vi "Example.vi"() -> ()   [LabVIEW 2014, in "Stanford Research DG645 - Driver.lvlib"]
uses:
  Stanford Research DG645 - Driver.lvlib
  Driver/Output BNC.ctl
  Driver/Channel.ctl
  Driver/Polarity.ctl
panel:
  in  "Main Tab Control":T1(tab)
  in  "Common IEEE-488.2 Tab Control":T2(tab)
  in  "Calibrate":bool
  out "Calibration Result Code":i32
  out "Auto Calibration passed succesfully":bool
  in  "Clear Status":bool
  out "Current ESE Register":i32
  in  "get ESE":bool
  in  "Set ESE Register":i32
  in  "get Event Status Register":bool
  out "Current Event Status Register Values":T3
  out "Current ESR Register":i32
  in  "Identify Device":bool
  out "Model":string
  out "Instrument Firmware Revision":string
  out "Complete Answer String":string
  out "Manufacturer":string
  out "Serial Number":string
  out "Operation complete?":bool
  out "Current Operation Comlete":i32
  in  "get Operation Complete":bool
  in  "set Operation Complete":bool
  out "Current PSC flag":bool
  in  "get PSC flag":bool
  in  "Set PSC flag":bool
  in  "Recall Settings":i32
  in  "Reset":bool
  in  "Save Settings":i32
  out "Current SRE":i32
  in  "get SRE":bool
  in  "Set SRE":i32
  in  "get Status Byte":bool
  out "Current Status Byte":i32
  out "Current Status Byte Register":T4
  in  "Trigger":bool
  in  "Self Test":bool
  out "Self-Test Result Code":i32
  out "Self Test passed succesfully":bool
  in  "Wait for Command Execution":bool
  in  "Status and Display":T5(tab)
  in  "Set Display Value":i32(ring) items=["Trigger rate", "Trigger threshold", "Trigger single shot", "Trigger line", "Advanced triggering enable", "Trigger holdoff", "Prescale configuration", "Burst mode", "Burst delay", "Burst count", "Burst period", "Channel delay", "Channel output levels", "Channel output polarity", "Burst T0 configuration"]
  in  "Set Channel":T6 items=["T0", "T1", "A", "B", "C", "D", "E", "F", "G", "H"]
  in  "Get Display":bool
  out "Current Display Value":i32(ring) items=["Trigger rate", "Trigger threshold", "Trigger single shot", "Trigger line", "Advanced triggering enable", "Trigger holdoff", "Prescale configuration", "Burst mode", "Burst delay", "Burst count", "Burst period", "Channel delay", "Channel output levels", "Channel output polarity", "Burst T0 configuration"]
  out "Current Channel":T6 items=["T0", "T1", "A", "B", "C", "D", "E", "F", "G", "H"]
  in  "Set INSE register":i32
  out "Current INSE register":i32
  in  "Get INSE register":bool
  in  "Get Instrument Status":bool
  out "Current Instrument Status Register Values":T7
  out "Current Instrument Status Register":i32
  in  "Get Error":bool
  in  "Set Show Display":bool
  out "Display shown?":bool
  in  "Get Show Display":bool
  in  "Get Timebase":bool
  out "Current Timebase":i32(ring) items=["Internal", "OCXO", "Rubidium", "External"]
  in  "Trigger":T8(tab)=enum."Step Holdoff"
  out "Adv. Trig. set?":bool
  in  "Set Adv. Triggering":bool
  in  "Get Adv. Triggering":bool
  out "Current Holdoff":dbl
  in  "Set Holdoff":dbl
  in  "Get Holdoff":bool
  in  "Set Inhibit":i32(ring) items=["Off", "Triggers", "AB", "AB and CD", "AB, CD and EF", "AB, CD, EF and GH"]
  in  "Get Inhibit":bool
  out "Current Trigger Inhibit State":i32(ring) items=["Off", "Triggers", "AB", "AB and CD", "AB, CD and EF", "AB, CD, EF and GH"]
  in  "Set Prescale Phase Factor":i32
  out "Current Prescale Phase Factor":i32
  in  "Prescaler to be set (PSPF)":i32(ring)=1 items=["Output AB"=1, "Output CD"=2, "Output EF"=3, "Output GH"=4]
  in  "Get Prescale Phase Factor":i32(ring)=1 items=["Output AB"=1, "Output CD"=2, "Output EF"=3, "Output GH"=4]
  in  "Set Prescale Factor":i32
  out "Current Prescale Factor":i32
  in  "Prescaler to be set (PSF)":i32(ring)=1 items=["Output AB"=1, "Output CD"=2, "Output EF"=3, "Output GH"=4]
  in  "Get Prescale Factor":i32(ring)=1 items=["Output AB"=1, "Output CD"=2, "Output EF"=3, "Output GH"=4]
  out "Step Size Holdoff [s]":dbl
  in  "Set Step Size Holdoff [s]":dbl
  in  "Holdoff Step Direction":bool
  in  "Step Holdoff":bool
  in  "Get Step Size Holdoff":bool
  out "Step Size Prescale Phase":i32
  in  "Set Step Size Prescale Phase":i32
  in  "Prescale Phase Step Direction":bool
  in  "Step Prescale Phase":bool
  in  "Get Step Size Prescale Phase":bool
  in  "Prescaler PPF":i32(ring)=1 items=["Output AB"=1, "Output CD"=2, "Output EF"=3, "Output GH"=4]
  out "Step Size  Phase Factor":i32
  in  "Set Step Size  Phase Factor":i32
  in  "Phase Factor Step Direction":bool
  in  "Step Phase Factor":bool
  in  "Get Step Size  Phase Factor":bool
  in  "Prescaler PF":i32(ring)=1 items=["Output AB"=1, "Output CD"=2, "Output EF"=3, "Output GH"=4]
  out "Step Size Trig Level [V]":dbl
  in  "Set Step Size Trig Level [V]":dbl
  in  "Trig Level Step Direction":bool
  in  "Step Trig Level":bool
  in  "Get Step Size Trig Level":bool
  out "Step Size Trig Rate [Hz]":dbl
  in  "Set Step Size Trig Rate [Hz]":dbl
  in  "Trig Rate Step Direction":bool
  in  "Step Trig Rate":bool
  in  "Get Step Size Trig Rate":bool
  in  "Get Trigger Level":bool
  in  "Set Trigger Level [V]":dbl=1.0
  out "Current Trigger Level [V]":dbl
  in  "Get Trigger Rate":bool
  in  "Set Trigger Rate [Hz]":dbl=1000.0
  out "Current Trigger Rate [Hz]":dbl
  in  "Set Trigger Source":i32(ring) items=["Internal", "External rising edge", "External falling edge", "Single shot external rising edges", "Single shot external falling edges", "Single shot", "Line"]
  in  "Get Trigger Source":bool
  out "Current Trigger Source":i32(ring) items=["Internal", "External rising edge", "External falling edge", "Single shot external rising edges", "Single shot external falling edges", "Single shot", "Line"]
  in  "Burst":T9(tab)
  out "Current Burst Count":i32
  in  "Set Burst Count":i32
  in  "Get Burst Count":bool
  out "Current Burst Delay [s]":dbl
  in  "Set Burst Delay [s]":dbl
  in  "Get Burst Delay":bool
  in  "Set Burst Mode":bool
  in  "Get Burst Mode":bool
  out "Burst Mode enabled?":bool
  in  "Set Burst Period [s]":dbl
  in  "Get Burst Period":bool
  out "Current Burst Period [s]":dbl
  in  "Set Burst T0 Config":bool
  in  "Get Burst T0 Config":bool
  out "Burst T0 Config enabled?":bool
  in  "Burst Count Step Direction":bool
  in  "Set Burst Count Step Size":i32
  in  "Step Burst Count":bool
  in  "Get Burst Count Step Size":bool
  out "Burst Count Step Size":i32
  in  "Burst Delay Step Direction":bool
  in  "Set Burst Delay Step Size [s]":dbl
  in  "Step Burst Delay":bool
  in  "Get Burst Delay Step Size":bool
  out "Burst Delay Step Size [s]":dbl
  in  "Burst Period Step Direction":bool
  in  "Set Burst Period Step Size [Hz]":dbl
  in  "Step Burst Period":bool
  in  "Get Burst Period Step Size":bool
  out "Burst Period Step Size [Hz]":dbl
  in  "Delay and Output":T10(tab)=enum."Offset"
  in  "Set: relative to":T6 items=["T0", "T1", "A", "B", "C", "D", "E", "F", "G", "H"]
  in  "Set: Delay [s]":dbl
  in  "Set Delay Channel":T6 items=["T0", "T1", "A", "B", "C", "D", "E", "F", "G", "H"]
  in  "Get Delay Channel":T6 items=["T0", "T1", "A", "B", "C", "D", "E", "F", "G", "H"]
  out "currently relative to":T6 items=["T0", "T1", "A", "B", "C", "D", "E", "F", "G", "H"]
  out "Current Delay [s]":dbl
  in  "Set: Level Amplitude [V]":dbl
  in  "Set Level Amplitude Output BNC":T11 items=["T0", "AB", "CD", "EF", "GH"]
  in  "Get Level Amplitude Output BNC":T11 items=["T0", "AB", "CD", "EF", "GH"]
  out "Current Level Amplitude Output BNC [V]":dbl
  in  "Set: Link to":T6=3 items=["T0", "T1", "A", "B", "C", "D", "E", "F", "G", "H"]
  in  "Set Link of Channel":T6=2 items=["T0", "T1", "A", "B", "C", "D", "E", "F", "G", "H"]
  in  "Get Link of Channel":T6=2 items=["T0", "T1", "A", "B", "C", "D", "E", "F", "G", "H"]
  out "currently linked to":T6 items=["T0", "T1", "A", "B", "C", "D", "E", "F", "G", "H"]
  in  "Set Level Offset [V]":dbl=1.0
  in  "Set Level Offset of Output":T11 items=["T0", "AB", "CD", "EF", "GH"]
  in  "Get Level Offset of Output":T11 items=["T0", "AB", "CD", "EF", "GH"]
  out "Current Level Offset [V]":dbl
  in  "Set Level Polarity of Output":T11 items=["T0", "AB", "CD", "EF", "GH"]
  in  "Get Level Polarity of Output":T11 items=["T0", "AB", "CD", "EF", "GH"]
  out "Current Polarity":T12 items=["negative", "positive"]
  in  "Polarity to be set":T12=1 items=["negative", "positive"]
  in  "Set Step Size Delay [s]":dbl
  in  "Delay Step Direction":bool
  in  "Step Delay":bool
  out "Step Size Delay [s]":dbl
  in  "Get Step Size Delay":bool
  in  "Channel Step Delay":T6 items=["T0", "T1", "A", "B", "C", "D", "E", "F", "G", "H"]
  in  "Set Step Size L-Amplitude [V]":dbl
  in  "Level Amplitude Step Direction":bool
  in  "Step Level Amplitude":bool
  out "Step Size  Level Amplitude [V]":dbl
  in  "Get Step Size Level Amplitude":bool
  in  "Output BNC Step Level Ampitude":T11 items=["T0", "AB", "CD", "EF", "GH"]
  in  "Set Step Size L-Offset [V]":dbl
  in  "Level Offset Step Direction":bool
  in  "Step Level Offset":bool
  out "Step Size  Level Offset [V]":dbl
  in  "Get Step Size Level Offset":bool
  in  "Output BNC Level Offset":T11 items=["T0", "AB", "CD", "EF", "GH"]
  in  "Interface":T13(tab)=enum."Interface Config"
  in  "Get Ethernet MAC Address":bool
  out "Ethernet MAC address":string="\r\n"
  out "Ethernet Physical Layer Config":bool
  in  "Get Ethernet Physical Layer Config":i32(ring) items=["Enable/disable Auto-negotiation of link speed", "Set link speed to 10 Base-T or 100 Base T"]
  in  "Set Ethernet Physical Layer Config":i32(ring) items=["Enable/disable Auto-negotiation of link speed", "Set link speed to 10 Base-T or 100 Base T"]
  in  "Ethernet Physical Layer Config to set":bool
  in  "Get Interface Config":i32(ring) items=["RS-232 Enable/Disable", "RS-232 Baud Rate", "GPIB Enable/Disable", "GPIB Address", "LAN TCP/IP Enable/Disable", "DHCP Enable/Disable", "Auto-Ip Enable/Disable", "Static Ip Enable/Disable", "Bare Socket Enable/Disable", "Telnet Enable/Disable", "VXI-11 Net Instrument Enable/Disable", "Static IP Address", "Subnet Address/Network Mask", "Default Gateway"]
  out "Current Interface Config Value":string
  in  "Set Interface Config":i32(ring) items=["RS-232 Enable/Disable", "RS-232 Baud Rate", "GPIB Enable/Disable", "GPIB Address", "LAN TCP/IP Enable/Disable", "DHCP Enable/Disable", "Auto-Ip Enable/Disable", "Static Ip Enable/Disable", "Bare Socket Enable/Disable", "Telnet Enable/Disable", "VXI-11 Net Instrument Enable/Disable", "Static IP Address", "Subnet Address/Network Mask", "Default Gateway"]
  in  "Interface Config Value to set":string
  in  "Interface to reset":i32(ring) items=["RS-232", "GPIB", "LAN TCP/IP"]
  in  "Set Local":bool
  in  "Set Remote":bool
  in  "Lock":bool
  out "locked?":bool
  out "unlocked?":bool
  in  "Unlock":bool
  in  "i":i32
  in  "j":i32
  in  "k":i32
  in  "Utility":enum32{"Revision"}(tab)
  in  "Get Revision":bool
  out "Instrument Driver Revision":string
  out "Instrument Firmware Rev":string
  out "Device Errors":cluster{"code":i32, "Text":string}[](array[cluster])
  in  "stop":bool
  out "error out":errorcluster
  in  "VISA resource name":refnum<visa-resource-name>
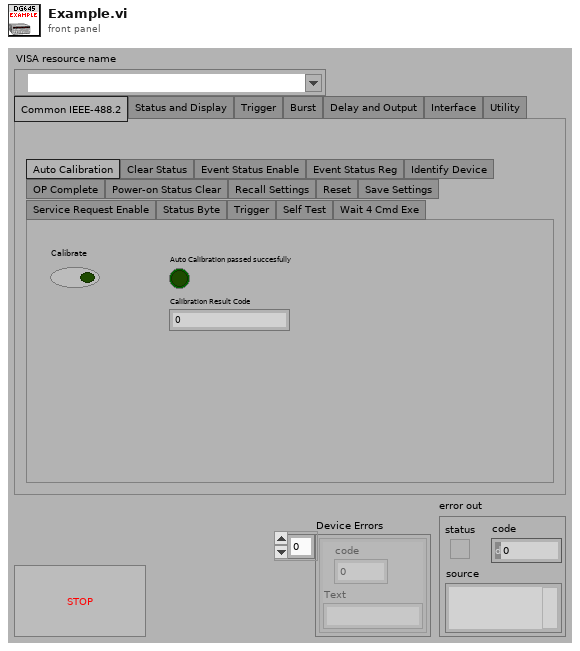
[diagram p1: front panel]
types:
  T1 = enum32{"Common IEEE-488.2", "Status and Display", "Trigger", "Burst", "Delay and Output", "Interface", "Utility"}
  T2 = enum32{"Auto Calibration", "Clear Status", "Event Status Enable", "Event Status Reg", "Identify Device", "OP Complete", "Power-on Status Clear", "Recall Settings", "Reset", "Save Settings", "Service Request Enable", "Status Byte", "Trigger", "Self Test", "Wait 4 Cmd Exe"}
  T3 = cluster{"Operation complete":bool, "reserved":bool, "Query Error":bool, "Device dependent Error":bool, "Execution Error":bool, "Command Error":bool, "reserved 2":bool, "Power-On":bool}
  T4 = cluster{"INSR Summary Bit":bool, "BUSY":bool, "reserved":bool, "reserved 2":bool, "message available":bool, "ESR Summary Bit":bool, "Master Summary Bit":bool, "reserved 3":bool}
  T5 = enum32{"Display", "Instrument Status Enable", "Instrument Status", "Error", "Show Display", "Timebase"}
  T6 = typedef "Stanford Research DG645 - Driver.lvlib/Channel.ctl" = i32
  T7 = cluster{"Got a trigger":bool, "Got a trigger while a delay or burst was in progress":bool, "a delay cycle has completed":bool, "a burst cycle has completed":bool, "a trigger or output delay cycle was inhibited":bool, "a delay cycle was aborted early":bool, "the 100MHz PLL came unlocked":bool, "the installed Rb oscillator is unlocked":bool}
  T8 = enum32{"Adv. Trig.", "Holdoff", "Inhibit", "Prescale Phase", "Prescale", "Step Holdoff", "Step PPF", "Step PF", "Step Trig Level", "Step Trig Rate", "Trig Level", "Trig Rate", "Trig Source"}
  T9 = enum32{"Count", "Delay", "Mode", "Period", "T0 Config", "Step Burst Count", "Step Burst Delay", "Step Bur Per"}
  T10 = enum32{"Delay", "Amplitude", "Link Channel", "Offset", "Polarity", "Step Delay", "Step Amplitude", "Step Offset"}
  T11 = typedef "Stanford Research DG645 - Driver.lvlib/Output BNC.ctl" = i32
  T12 = typedef "Stanford Research DG645 - Driver.lvlib/Polarity.ctl" = i32
  T13 = enum32{"MAC", "Ethernet Config", "Interface Config", "Interface Reset", "Local/Remote", "Lock/Unlock", "Term"}
  T14 = typedef "Stanford Research DG645.lvlib/Channel.ctl" = i32
  T15 = typedef "Stanford Research DG645.lvlib/Output BNC.ctl" = i32
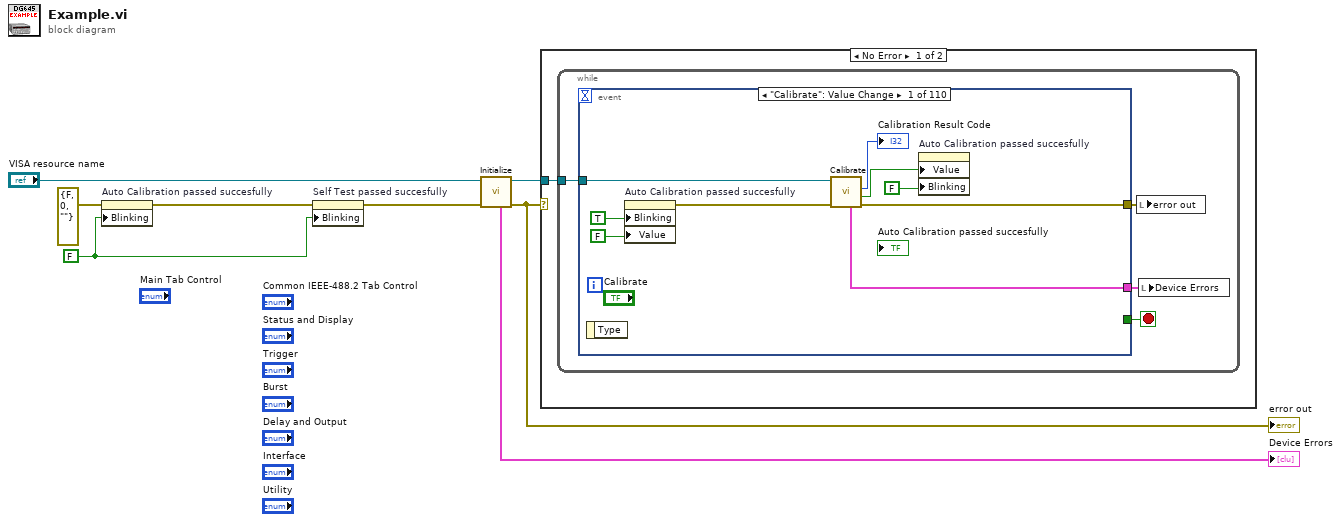
[diagram p0: block diagram]
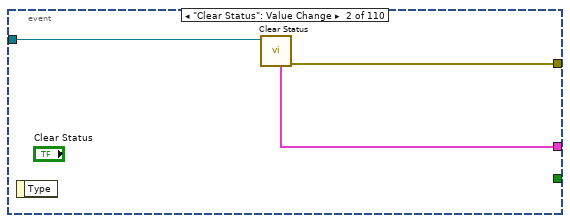
[diagram p2: hidden frame]
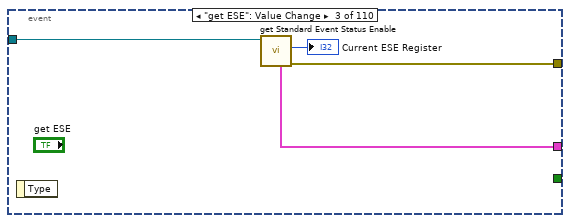
[diagram p3: hidden frame]
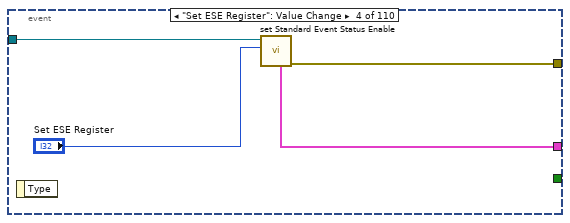
[diagram p4: hidden frame]
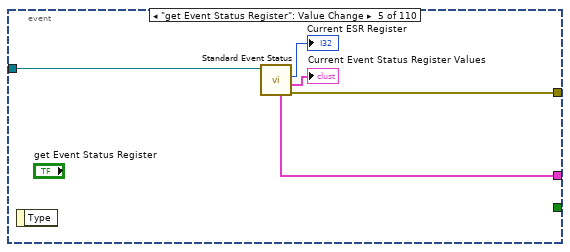
[diagram p5: hidden frame]
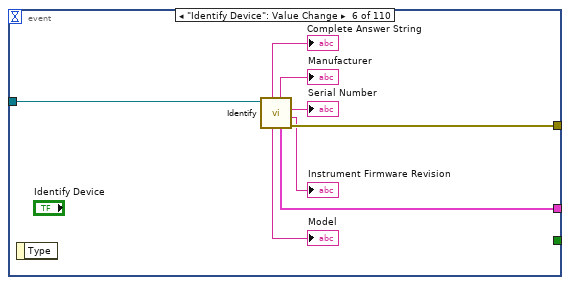
[diagram p6: hidden frame]
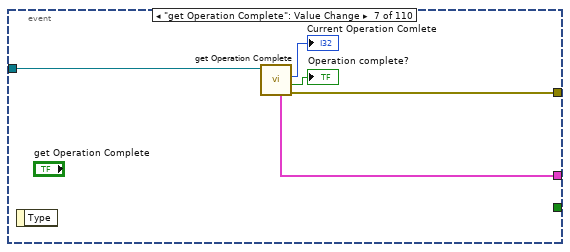
[diagram p7: hidden frame]
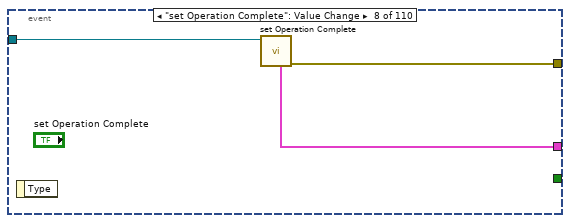
[diagram p8: hidden frame]
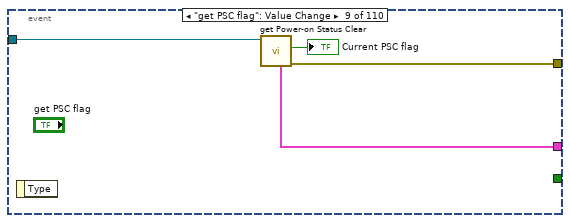
[diagram p9: hidden frame]
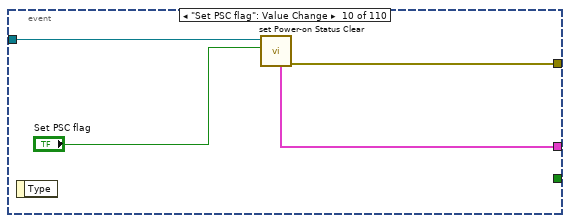
[diagram p10: hidden frame]
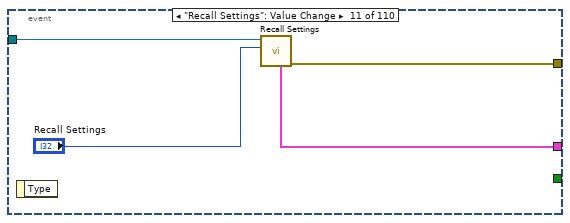
[diagram p11: hidden frame]
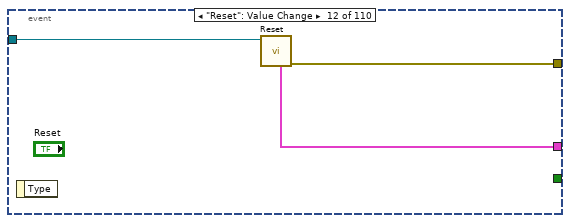
[diagram p12: hidden frame]
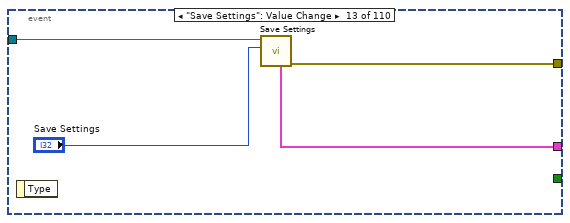
[diagram p13: hidden frame]
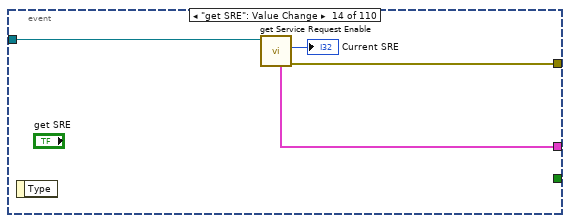
[diagram p14: hidden frame]
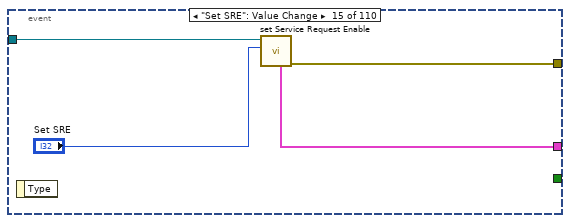
[diagram p15: hidden frame]
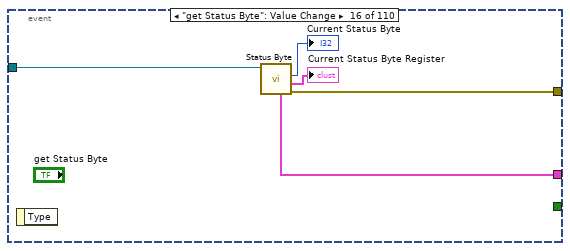
[diagram p16: hidden frame]
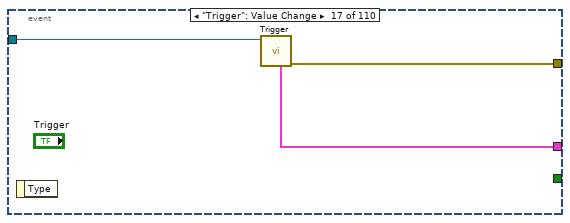
[diagram p17: hidden frame]
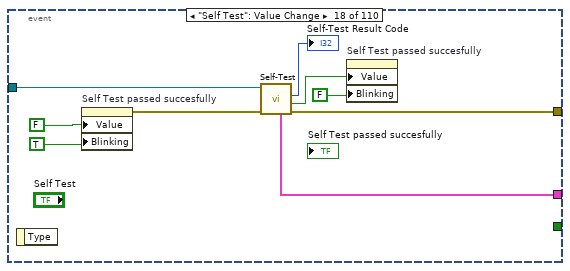
[diagram p18: hidden frame]
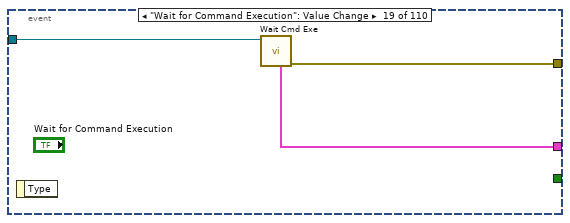
[diagram p19: hidden frame]
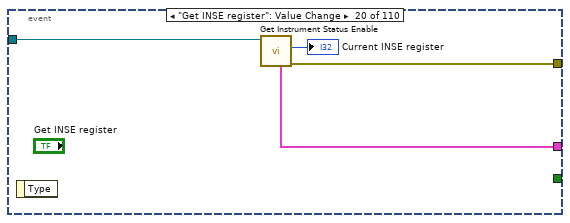
[diagram p20: hidden frame]
diagram:
  w1 = FALSE
  n1 = property on="Auto Calibration passed succesfully" class="Bool (strict)"(error in=errorcluster {"status"=FALSE, "code"=0, "source"=""} ("error out"), "Blinking"=w1) -> (error out=w4:errorcluster)  [unwired: 1 in, 1 out]
  n2 = property on="Self Test passed succesfully" class="Bool (strict)"(error in=w4, "Blinking"=w1) -> (error out=w2:errorcluster)  [unwired: 1 in, 1 out]
  n3 = call "Initialize.vi"("error in (no error)"=w2, "VISA resource name"="VISA resource name") -> ("error out"=w6:errorcluster, "VISA resource name out"=w7:refnum<visa-resource-name>, "Device Errors"=→"Device Errors":cluster{"code":i32, "Text":string}[])  [unwired: 7 in]
  "error out" <- w6
  n4 = case shown="No Error" w6 {
    tunnel: w7 -> [w9 _]
    frame No Error {
      n5 = while {
        tunnel: w9 -> [w13]
        stop <- w12 stop-if-true
        n6 = event shown="[0] \"Calibrate\": Value Change" {
          selector: _ -> [_ _ _ _ _ _ _ _ _ _ _ _ _ _ _ _ _ _ _ _ _ _ _ _ _ _ _ _ _ _ _ _ _ _ _ _ _ _ _ _ _ _ _ _ _ _ _ _ _ _ _ _ _ _ _ _ _ _ _ _ _ _ _ _ _ _ _ _ _ _ _ _ _ _ _ _ _ _ _ _ _ _ _ _ _ _ _ _ _ _ _ _ _ _ _ _ _ _ _ _ _ _ _ _ _ _ _ _ _ _]
          dyn-events: _ -> [_ _ _ _ _ _ _ _ _ _ _ _ _ _ _ _ _ _ _ _ _ _ _ _ _ _ _ _ _ _ _ _ _ _ _ _ _ _ _ _ _ _ _ _ _ _ _ _ _ _ _ _ _ _ _ _ _ _ _ _ _ _ _ _ _ _ _ _ _ _ _ _ _ _ _ _ _ _ _ _ _ _ _ _ _ _ _ _ _ _ _ _ _ _ _ _ _ _ _ _ _ _ _ _ _ _ _ _ _ _]
          timeout: _ -> [_ _ _ _ _ _ _ _ _ _ _ _ _ _ _ _ _ _ _ _ _ _ _ _ _ _ _ _ _ _ _ _ _ _ _ _ _ _ _ _ _ _ _ _ _ _ _ _ _ _ _ _ _ _ _ _ _ _ _ _ _ _ _ _ _ _ _ _ _ _ _ _ _ _ _ _ _ _ _ _ _ _ _ _ _ _ _ _ _ _ _ _ _ _ _ _ _ _ _ _ _ _ _ _ _ _ _ _ _ _]
          tunnel: [w14 w25 w29 w33 w38 w46 w51 w54 w58 w62 w66 w69 w73 w77 w81 w86 w87 w90 w99 w103 w108 w113 w117 w122 w127 w131 w135 w139 w143 w147 w151 w155 w159 w163 w168 w173 w177 w182 w186 w190 w194 w199 w205 w211 w216 w222 w228 w232 w236 w240 w244 w248 w252 w256 w260 w264 w268 w272 w276 w280 w284 w288 w292 w296 w300 w304 w308 w312 w316 w320 w324 w328 w332 w336 w340 w344 w348 w352 w358 w364 w369 w374 w379 w384 w389 w394 w399 w404 w409 w415 w421 w426 w432 w438 w443 w449 w455 w459 w464 w469 w474 w479 w483 w486 w490 w493 w497 w503 w508 w512] -> w11
          tunnel: w13 -> [w22 w24 w28 w32 w37 w45 w50 w53 w57 w61 w65 w68 w72 w76 w80 w85 w89 w98 w101 w105 w110 w115 w119 w124 w126 w130 w134 w138 w142 w146 w150 w154 w158 w162 w167 w172 w176 w181 w185 w189 w193 w198 w204 w210 w215 w221 w227 w231 w235 w239 w243 w247 w251 w255 w259 w263 w267 w271 w275 w279 w283 w287 w291 w295 w299 w303 w307 w311 w315 w319 w323 w327 w331 w335 w339 w343 w347 w351 w357 w363 w368 w373 w378 w383 w388 w393 w398 w403 w408 w414 w420 w425 w431 w437 w442 w448 w454 w458 w463 w468 w473 w478 w482 w485 w489 w492 w496 w502 w507 w511]
          tunnel: [_ _ _ _ _ _ _ _ _ _ _ _ _ _ _ _ _ _ _ _ _ _ _ _ _ _ _ _ _ _ _ _ _ _ _ _ _ _ _ _ _ _ _ _ _ _ _ _ _ _ _ _ _ _ _ _ _ _ _ _ _ _ _ _ _ _ _ _ _ _ _ _ _ _ _ _ _ _ _ _ _ _ _ _ _ _ _ _ _ _ _ _ _ _ _ _ _ _ _ _ _ _ _ _ _ _ _ _ _ "stop"] -> w12
          tunnel: [w21 w23 w27 w31 w36 w44 w49 w52 w56 w60 w64 w67 w71 w75 w79 w84 w88 w97 w100 w104 w109 w114 w118 w123 w125 w129 w133 w137 w141 w145 w149 w153 w157 w161 w166 w171 w175 w180 w184 w188 w192 w197 w203 w209 w214 w220 w226 w230 w234 w238 w242 w246 w250 w254 w258 w262 w266 w270 w274 w278 w282 w286 w290 w294 w298 w302 w306 w310 w314 w318 w322 w326 w330 w334 w338 w342 w346 w350 w356 w362 w367 w372 w377 w382 w387 w392 w397 w402 w407 w413 w419 w424 w430 w436 w441 w447 w453 w457 w462 w467 w472 w477 w481 w484 w488 w491 w495 w501 w506 w509] -> w10
          event "Calibrate": Value Change {
            n7 = event-data() -> ()  [unwired: 1 in, 1 out]
            n8 = property on="Auto Calibration passed succesfully" class="Bool (strict)"("Blinking"=TRUE, "Value"=FALSE ("Auto Calibration passed succesfully")) -> (error out=w19:errorcluster)  [unwired: 2 in, 1 out]
            n9 = call "Calibrate.vi"("error in (no error)"=w19, "VISA resource name"=w22) -> ("error out"=w14:errorcluster, "Auto Calibration successful"=w15:bool, "Calibtration Result Code"=→"Calibration Result Code":i32, "Device Errors"=w21:cluster{"code":i32, "Text":string}[])  [unwired: 5 in, 1 out]
            n10 = property on="Auto Calibration passed succesfully" class="Bool (strict)"("Value"=w15, "Blinking"=FALSE) -> ()  [unwired: 2 in, 2 out]
          }
          event "Clear Status": Value Change {
            n11 = event-data() -> ()  [unwired: 1 in, 1 out]
            n12 = call "Clear Status.vi"("VISA resource name"=w24) -> ("error out"=w25:errorcluster, "Device Errors"=w23:cluster{"code":i32, "Text":string}[])  [unwired: 8 in, 1 out]
          }
          event "get ESE": Value Change {
            n13 = event-data() -> ()  [unwired: 1 in, 1 out]
            n14 = call "get Standard Event Status Enable.vi"("VISA resource name"=w28) -> ("error out"=w29:errorcluster, "ESE register"=→"Current ESE Register":i32, "Device Errors"=w27:cluster{"code":i32, "Text":string}[])  [unwired: 7 in, 1 out]
          }
          event "Set ESE Register": Value Change {
            n15 = event-data() -> ()  [unwired: 1 in, 1 out]
            n16 = call "set Standard Event Status Enable.vi"("Value ESE register (0)"="Set ESE Register", "VISA resource name"=w32) -> ("error out"=w33:errorcluster, "Device Errors"=w31:cluster{"code":i32, "Text":string}[])  [unwired: 7 in, 1 out]
          }
          event "get Event Status Register": Value Change {
            n17 = event-data() -> ()  [unwired: 1 in, 1 out]
            n18 = call "Standard Event Status.vi"("VISA resource name"=w37) -> ("error out"=w38:errorcluster, "Event Status Register Values"=→"Current Event Status Register Values":T3, "ESR register"=→"Current ESR Register":i32, "Device Errors"=w36:cluster{"code":i32, "Text":string}[])  [unwired: 6 in, 1 out]
          }
          event "Identify Device": Value Change {
            n19 = event-data() -> ()  [unwired: 1 in, 1 out]
            n20 = call "Identify.vi"("VISA resource name"=w45) -> ("error out"=w46:errorcluster, "Instrument Firmware Revision"=→"Instrument Firmware Revision":string, "Serial Number"=→"Serial Number":string, "Device Errors"=w44:cluster{"code":i32, "Text":string}[], "Manufacturer"=→"Manufacturer":string, "Model"=→"Model":string, "Instrument identification string"=→"Complete Answer String":string)  [unwired: 3 in, 1 out]
          }
          event "get Operation Complete": Value Change {
            n21 = event-data() -> ()  [unwired: 1 in, 1 out]
            n22 = call "get Operation Complete.vi"("VISA resource name"=w50) -> ("error out"=w51:errorcluster, "Operation complete?"=→"Operation complete?":bool, "Result"=→"Current Operation Comlete":i32, "Device Errors"=w49:cluster{"code":i32, "Text":string}[])  [unwired: 6 in, 1 out]
          }
          event "set Operation Complete": Value Change {
            n23 = event-data() -> ()  [unwired: 1 in, 1 out]
            n24 = call "set Operation Complete.vi"("VISA resource name"=w53) -> ("error out"=w54:errorcluster, "Device Errors"=w52:cluster{"code":i32, "Text":string}[])  [unwired: 8 in, 1 out]
          }
          event "get PSC flag": Value Change {
            n25 = event-data() -> ()  [unwired: 1 in, 1 out]
            n26 = call "get Power-on Status Clear.vi"("VISA resource name"=w57) -> ("error out"=w58:errorcluster, "Power-on Status Flag"=→"Current PSC flag":bool, "Device Errors"=w56:cluster{"code":i32, "Text":string}[])  [unwired: 7 in, 1 out]
          }
          event "Set PSC flag": Value Change {
            n27 = event-data() -> ()  [unwired: 1 in, 1 out]
            n28 = call "set Power-on Status Clear.vi"("PSC Flag (false)"="Set PSC flag", "VISA resource name"=w61) -> ("error out"=w62:errorcluster, "Device Errors"=w60:cluster{"code":i32, "Text":string}[])  [unwired: 7 in, 1 out]
          }
          event "Recall Settings": Value Change {
            n29 = event-data() -> ()  [unwired: 1 in, 1 out]
            n30 = call "Recall Settings.vi"("Location (0)"="Recall Settings", "VISA resource name"=w65) -> ("error out"=w66:errorcluster, "Device Errors"=w64:cluster{"code":i32, "Text":string}[])  [unwired: 7 in, 1 out]
          }
          event "Reset": Value Change {
            n31 = event-data() -> ()  [unwired: 1 in, 1 out]
            n32 = call "Reset.vi"("VISA resource name"=w68) -> ("error out"=w69:errorcluster, "Device Errors"=w67:cluster{"code":i32, "Text":string}[])  [unwired: 8 in, 1 out]
          }
          event "Save Settings": Value Change {
            n33 = event-data() -> ()  [unwired: 1 in, 1 out]
            n34 = call "Save Settings.vi"("Location (0)"="Save Settings", "VISA resource name"=w72) -> ("error out"=w73:errorcluster, "Device Errors"=w71:cluster{"code":i32, "Text":string}[])  [unwired: 7 in, 1 out]
          }
          event "get SRE": Value Change {
            n35 = event-data() -> ()  [unwired: 1 in, 1 out]
            n36 = call "get Service Request Enable.vi"("VISA resource name"=w76) -> ("error out"=w77:errorcluster, "SRE register"=→"Current SRE":i32, "Device Errors"=w75:cluster{"code":i32, "Text":string}[])  [unwired: 7 in, 1 out]
          }
          event "Set SRE": Value Change {
            n37 = event-data() -> ()  [unwired: 1 in, 1 out]
            n38 = call "set Service Request Enable.vi"("Value SRE register (0)"="Set SRE", "VISA resource name"=w80) -> ("error out"=w81:errorcluster, "Device Errors"=w79:cluster{"code":i32, "Text":string}[])  [unwired: 7 in, 1 out]
          }
          event "get Status Byte": Value Change {
            n39 = event-data() -> ()  [unwired: 1 in, 1 out]
            n40 = call "Status Byte.vi"("VISA resource name"=w85) -> ("error out"=w86:errorcluster, "Status Byte Register Values"=→"Current Status Byte Register":T4, "Status Byte"=→"Current Status Byte":i32, "Device Errors"=w84:cluster{"code":i32, "Text":string}[])  [unwired: 6 in, 1 out]
          }
          event "Trigger": Value Change {
            n41 = event-data() -> ()  [unwired: 1 in, 1 out]
            n42 = call "Trigger.vi"("VISA resource name"=w89) -> ("error out"=w87:errorcluster, "Device Errors"=w88:cluster{"code":i32, "Text":string}[])  [unwired: 8 in, 1 out]
          }
          event "Self Test": Value Change {
            n43 = event-data() -> ()  [unwired: 1 in, 1 out]
            n44 = property on="Self Test passed succesfully" class="Bool (strict)"("Value"=FALSE ("Self Test passed succesfully"), "Blinking"=TRUE) -> (error out=w95:errorcluster)  [unwired: 2 in, 1 out]
            n45 = call "Self-Test.vi"("error in (no error)"=w95, "VISA resource name"=w98) -> ("error out"=w90:errorcluster, "Self Test successful"=w91:bool, "Self-Test Result Code"=→"Self-Test Result Code":i32, "Device Errors"=w97:cluster{"code":i32, "Text":string}[])  [unwired: 5 in, 1 out]
            n46 = property on="Self Test passed succesfully" class="Bool (strict)"("Value"=w91, "Blinking"=FALSE) -> ()  [unwired: 2 in, 2 out]
          }
          event "Wait for Command Execution": Value Change {
            n47 = event-data() -> ()  [unwired: 1 in, 1 out]
            n48 = call "Wait Cmd Exe.vi"("VISA resource name"=w101) -> ("error out"=w99:errorcluster, "Device Errors"=w100:cluster{"code":i32, "Text":string}[])  [unwired: 8 in, 1 out]
          }
          event "Get INSE register": Value Change {
            n49 = event-data() -> ()  [unwired: 1 in, 1 out]
            n50 = call "Get Instrument Status Enable.vi"("VISA resource name"=w105) -> ("error out"=w103:errorcluster, "INSE register"=→"Current INSE register":i32, "Device Errors"=w104:cluster{"code":i32, "Text":string}[])  [unwired: 7 in, 1 out]
          }
          event "Get Display": Value Change {
            n51 = event-data() -> ()  [unwired: 1 in, 1 out]
            n52 = call "Get Display.vi"("VISA resource name"=w110) -> ("error out"=w108:errorcluster, "Channel"=→"Current Channel":T6, "Display Value"=→"Current Display Value":i32, "Device Errors"=w109:cluster{"code":i32, "Text":string}[])  [unwired: 6 in, 1 out]
          }
          event "Set Display Value": Value Change {
            n53 = event-data() -> ()  [unwired: 1 in, 1 out]
            n54 = call "Set Display.vi"("Channel (T0)"="Set Channel", "Display Value (Trigger Rate)"="Set Display Value", "VISA resource name"=w115) -> ("error out"=w113:errorcluster, "Device Errors"=w114:cluster{"code":i32, "Text":string}[])  [unwired: 6 in, 1 out]
          }
          event "Set INSE register": Value Change {
            n55 = event-data() -> ()  [unwired: 1 in, 1 out]
            n56 = call "Set Instrument Status Enable.vi"("INSE (0)"="Set INSE register", "VISA resource name"=w119) -> ("error out"=w117:errorcluster, "Device Errors"=w118:cluster{"code":i32, "Text":string}[])  [unwired: 7 in, 1 out]
          }
          event "Get Instrument Status": Value Change {
            n57 = event-data() -> ()  [unwired: 1 in, 1 out]
            n58 = call "Instrument Status Register.vi"("VISA resource name"=w124) -> ("error out"=w122:errorcluster, "Instrument Status Register Values"=→"Current Instrument Status Register Values":T7, "Instrument Status Register"=→"Current Instrument Status Register":i32, "Device Errors"=w123:cluster{"code":i32, "Text":string}[])  [unwired: 6 in, 1 out]
          }
          event "Get Error": Value Change {
            n59 = event-data() -> ()  [unwired: 1 in, 1 out]
            n60 = call "Error Query.vi"("VISA resource name"=w126) -> ("error out"=w127:errorcluster, "Device Errors"=w125:cluster{"code":i32, "Text":string}[])  [unwired: 8 in, 1 out]
          }
          event "Get Show Display": Value Change {
            n61 = event-data() -> ()  [unwired: 1 in, 1 out]
            n62 = call "Get Show Display.vi"("VISA resource name"=w130) -> ("error out"=w131:errorcluster, "Display on?"=→"Display shown?":bool, "Device Errors"=w129:cluster{"code":i32, "Text":string}[])  [unwired: 7 in, 1 out]
          }
          event "Set Show Display": Value Change {
            n63 = event-data() -> ()  [unwired: 1 in, 1 out]
            n64 = call "Set Show Display.vi"("Show Display (true)"="Set Show Display", "VISA resource name"=w134) -> ("error out"=w135:errorcluster, "Device Errors"=w133:cluster{"code":i32, "Text":string}[])  [unwired: 7 in, 1 out]
          }
          event "Get Timebase": Value Change {
            n65 = event-data() -> ()  [unwired: 1 in, 1 out]
            n66 = call "Timebase.vi"("VISA resource name"=w138) -> ("error out"=w139:errorcluster, "Timebase"=→"Current Timebase":i32, "Device Errors"=w137:cluster{"code":i32, "Text":string}[])  [unwired: 7 in, 1 out]
          }
          event "Get Adv. Triggering": Value Change {
            n67 = event-data() -> ()  [unwired: 1 in, 1 out]
            n68 = call "Get Advanced Triggering Mode.vi"("VISA resource name"=w142) -> ("error out"=w143:errorcluster, "Adv Trig Mode enabled?"=→"Adv. Trig. set?":bool, "Device Errors"=w141:cluster{"code":i32, "Text":string}[])  [unwired: 7 in, 1 out]
          }
          event "Set Adv. Triggering": Value Change {
            n69 = event-data() -> ()  [unwired: 1 in, 1 out]
            n70 = call "Set Advanced Triggering Mode.vi"("Enable Adv Trig Mode"="Set Adv. Triggering", "VISA resource name"=w146) -> ("error out"=w147:errorcluster, "Device Errors"=w145:cluster{"code":i32, "Text":string}[])  [unwired: 7 in, 1 out]
          }
          event "Get Holdoff": Value Change {
            n71 = event-data() -> ()  [unwired: 1 in, 1 out]
            n72 = call "Get Holdoff.vi"("VISA resource name"=w150) -> ("error out"=w151:errorcluster, "Holdoff [s]"=→"Current Holdoff":dbl, "Device Errors"=w149:cluster{"code":i32, "Text":string}[])  [unwired: 7 in, 1 out]
          }
          event "Set Holdoff": Value Change {
            n73 = event-data() -> ()  [unwired: 1 in, 1 out]
            n74 = call "Set Holdoff.vi"("Holdoff (0) [s]"="Set Holdoff", "VISA resource name"=w154) -> ("error out"=w155:errorcluster, "Device Errors"=w153:cluster{"code":i32, "Text":string}[])  [unwired: 7 in, 1 out]
          }
          event "Get Inhibit": Value Change {
            n75 = event-data() -> ()  [unwired: 1 in, 1 out]
            n76 = call "Get Inhibit.vi"("VISA resource name"=w158) -> ("error out"=w159:errorcluster, "Inhibit"=→"Current Trigger Inhibit State":i32, "Device Errors"=w157:cluster{"code":i32, "Text":string}[])  [unwired: 7 in, 1 out]
          }
          event "Set Inhibit": Value Change {
            n77 = event-data() -> ()  [unwired: 1 in, 1 out]
            n78 = call "Set Inhibit.vi"("Inhibit (Off)"="Set Inhibit", "VISA resource name"=w162) -> ("error out"=w163:errorcluster, "Device Errors"=w161:cluster{"code":i32, "Text":string}[])  [unwired: 7 in, 1 out]
          }
          event "Get Prescale Phase Factor": Value Change {
            n79 = event-data() -> ()  [unwired: 1 in, 1 out]
            n80 = call "Get Prescale Phase Factor.vi"("Prescaler (Output AB)"="Get Prescale Phase Factor", "VISA resource name"=w167) -> ("error out"=w168:errorcluster, "Prescale Phase Factor"=→"Current Prescale Phase Factor":i32, "Device Errors"=w166:cluster{"code":i32, "Text":string}[])  [unwired: 6 in, 1 out]
          }
          event "Set Prescale Phase Factor", "Prescaler to be set (PSPF)": Value Change {
            n81 = event-data() -> ()  [unwired: 1 in, 1 out]
            n82 = call "Set Prescale Phase Factor.vi"("Prescale Phase Factor (0)"="Set Prescale Phase Factor", "Prescaler (Output AB)"="Prescaler to be set (PSPF)", "VISA resource name"=w172) -> ("error out"=w173:errorcluster, "Device Errors"=w171:cluster{"code":i32, "Text":string}[])  [unwired: 6 in, 1 out]
          }
          event "Get Prescale Factor": Value Change {
            n83 = event-data() -> ()  [unwired: 1 in, 1 out]
            n84 = call "Get Prescale Factor.vi"("VISA resource name"=w176) -> ("error out"=w177:errorcluster, "Prescale Factor"=→"Current Prescale Factor":i32, "Device Errors"=w175:cluster{"code":i32, "Text":string}[])  [unwired: 7 in, 1 out]
          }
          event "Prescaler to be set (PSF)": Value Change {
            n85 = event-data() -> ()  [unwired: 1 in, 1 out]
            n86 = call "Set Prescale Factor.vi"("Prescale Factor (0)"="Set Prescale Factor", "Prescaler (Trigger Input)"="Prescaler to be set (PSF)", "VISA resource name"=w181) -> ("error out"=w182:errorcluster, "Device Errors"=w180:cluster{"code":i32, "Text":string}[])  [unwired: 6 in, 1 out]
          }
          event "Step Holdoff": Value Change {
            n87 = event-data() -> ()  [unwired: 1 in, 1 out]
            n88 = call "Step Holdoff.vi"("Step up? (false)"="Holdoff Step Direction", "VISA resource name"=w185) -> ("error out"=w186:errorcluster, "Device Errors"=w184:cluster{"code":i32, "Text":string}[])  [unwired: 7 in, 1 out]
          }
          event "Get Step Size Holdoff": Value Change {
            n89 = event-data() -> ()  [unwired: 1 in, 1 out]
            n90 = call "Get Step Size Holdoff.vi"("VISA resource name"=w189) -> ("error out"=w190:errorcluster, "Step Size Holdoff [s]"=→"Step Size Holdoff [s]":dbl, "Device Errors"=w188:cluster{"code":i32, "Text":string}[])  [unwired: 7 in, 1 out]
          }
          event "Set Step Size Holdoff [s]": Value Change {
            n91 = event-data() -> ()  [unwired: 1 in, 1 out]
            n92 = call "Set Step Size Holdoff.vi"("Step Size Holdoff (1) [s]"="Set Step Size Holdoff [s]", "VISA resource name"=w193) -> ("error out"=w194:errorcluster, "Device Errors"=w192:cluster{"code":i32, "Text":string}[])  [unwired: 7 in, 1 out]
          }
          event "Step Prescale Phase": Value Change {
            n93 = event-data() -> ()  [unwired: 1 in, 1 out]
            n94 = call "Step Prescale Phase Factor.vi"("Step up? (false)"="Prescale Phase Step Direction", "Prescaler (Output AB)"="Prescaler PPF", "VISA resource name"=w198) -> ("error out"=w199:errorcluster, "Device Errors"=w197:cluster{"code":i32, "Text":string}[])  [unwired: 6 in, 1 out]
          }
          event "Get Step Size Prescale Phase": Value Change {
            n95 = event-data() -> ()  [unwired: 1 in, 1 out]
            n96 = property on="Prescaler PPF" class="Ring (strict)"() -> (error out=w200:errorcluster, "Value"=w201:i32)  [unwired: 2 in, 1 out]
            n97 = call "Get Step Size Prescale Phase Factor.vi"("error in (no error)"=w200, "Prescaler (Output AB)"=w201, "VISA resource name"=w204) -> ("error out"=w205:errorcluster, "Step Size Prescale Phase Factor"=→"Step Size Prescale Phase":i32, "Device Errors"=w203:cluster{"code":i32, "Text":string}[])  [unwired: 5 in, 1 out]
          }
          event "Set Step Size Prescale Phase": Value Change {
            n98 = event-data() -> ()  [unwired: 1 in, 1 out]
            n99 = property on="Prescaler PPF" class="Ring (strict)"() -> (error out=w206:errorcluster, "Value"=w207:i32)  [unwired: 2 in, 1 out]
            n100 = call "Set Step Size Prescale Phase Factor.vi"("error in (no error)"=w206, "Step Size Prescale Phase Factor (1)"="Set Step Size Prescale Phase", "Prescaler (Output AB)"=w207, "VISA resource name"=w210) -> ("error out"=w211:errorcluster, "Device Errors"=w209:cluster{"code":i32, "Text":string}[])  [unwired: 5 in, 1 out]
          }
          event "Step Phase Factor": Value Change {
            n101 = event-data() -> ()  [unwired: 1 in, 1 out]
            n102 = call "Step Prescale Factor.vi"("Step up? (false)"="Phase Factor Step Direction", "Prescaler (Trigger Input)"="Prescaler PF", "VISA resource name"=w215) -> ("error out"=w216:errorcluster, "Device Errors"=w214:cluster{"code":i32, "Text":string}[])  [unwired: 6 in, 1 out]
          }
          event "Get Step Size  Phase Factor": Value Change {
            n103 = event-data() -> ()  [unwired: 1 in, 1 out]
            n104 = property on="Prescaler PF" class="Ring (strict)"() -> (error out=w218:errorcluster, "Value"=w217:i32)  [unwired: 2 in, 1 out]
            n105 = call "Get Prescale Factor.vi"("error in (no error)"=w218, "Prescaler (Trigger input)"=w217, "VISA resource name"=w221) -> ("error out"=w222:errorcluster, "Prescale Factor"=→"Step Size  Phase Factor":i32, "Device Errors"=w220:cluster{"code":i32, "Text":string}[])  [unwired: 5 in, 1 out]
          }
          event "Set Step Size  Phase Factor": Value Change {
            n106 = event-data() -> ()  [unwired: 1 in, 1 out]
            n107 = property on="Prescaler PF" class="Ring (strict)"() -> (error out=w225:errorcluster, "Value"=w224:i32)  [unwired: 2 in, 1 out]
            n108 = call "Set Step Size Prescale Factor.vi"("error in (no error)"=w225, "Step Size Prescale Factor (1)"="Set Step Size  Phase Factor", "Prescaler (Trigger Input)"=w224, "VISA resource name"=w227) -> ("error out"=w228:errorcluster, "Device Errors"=w226:cluster{"code":i32, "Text":string}[])  [unwired: 5 in, 1 out]
          }
          event "Step Trig Level": Value Change {
            n109 = event-data() -> ()  [unwired: 1 in, 1 out]
            n110 = call "Step Trigger Level.vi"("Step up? (false)"="Trig Level Step Direction", "VISA resource name"=w231) -> ("error out"=w232:errorcluster, "Device Errors"=w230:cluster{"code":i32, "Text":string}[])  [unwired: 7 in, 1 out]
          }
          event "Get Step Size Trig Level": Value Change {
            n111 = event-data() -> ()  [unwired: 1 in, 1 out]
            n112 = call "Get Step Size Trigger Level.vi"("VISA resource name"=w235) -> ("error out"=w236:errorcluster, "Step Size Trigger Level [V]"=→"Step Size Trig Level [V]":dbl, "Device Errors"=w234:cluster{"code":i32, "Text":string}[])  [unwired: 7 in, 1 out]
          }
          event "Set Step Size Trig Level [V]": Value Change {
            n113 = event-data() -> ()  [unwired: 1 in, 1 out]
            n114 = call "Set Step Size Trigger Level.vi"("Step Size Trigger Level (0.1) [V]"="Set Step Size Trig Level [V]", "VISA resource name"=w239) -> ("error out"=w240:errorcluster, "Device Errors"=w238:cluster{"code":i32, "Text":string}[])  [unwired: 7 in, 1 out]
          }
          event "Step Trig Rate": Value Change {
            n115 = event-data() -> ()  [unwired: 1 in, 1 out]
            n116 = call "Step Trigger Rate.vi"("Step up? (false)"="Trig Rate Step Direction", "VISA resource name"=w243) -> ("error out"=w244:errorcluster, "Device Errors"=w242:cluster{"code":i32, "Text":string}[])  [unwired: 7 in, 1 out]
          }
          event "Get Step Size Trig Rate": Value Change {
            n117 = event-data() -> ()  [unwired: 1 in, 1 out]
            n118 = call "Get Step Size Trigger Rate.vi"("VISA resource name"=w247) -> ("error out"=w248:errorcluster, "Step Size Trigger Rate [Hz]"=→"Step Size Trig Rate [Hz]":dbl, "Device Errors"=w246:cluster{"code":i32, "Text":string}[])  [unwired: 7 in, 1 out]
          }
          event "Set Step Size Trig Rate [Hz]": Value Change {
            n119 = event-data() -> ()  [unwired: 1 in, 1 out]
            n120 = call "Set Step Size Trigger Rate.vi"("Step Size Trigger Rate (10) [Hz]"="Set Step Size Trig Rate [Hz]", "VISA resource name"=w251) -> ("error out"=w252:errorcluster, "Device Errors"=w250:cluster{"code":i32, "Text":string}[])  [unwired: 7 in, 1 out]
          }
          event "Get Trigger Level": Value Change {
            n121 = event-data() -> ()  [unwired: 1 in, 1 out]
            n122 = call "Get Trigger Level.vi"("VISA resource name"=w255) -> ("error out"=w256:errorcluster, "Trigger Level [V]"=→"Current Trigger Level [V]":dbl, "Device Errors"=w254:cluster{"code":i32, "Text":string}[])  [unwired: 7 in, 1 out]
          }
          event "Set Trigger Level [V]": Value Change {
            n123 = event-data() -> ()  [unwired: 1 in, 1 out]
            n124 = call "Set Trigger Level.vi"("Trigger Level (1) [V]"="Set Trigger Level [V]", "VISA resource name"=w259) -> ("error out"=w260:errorcluster, "Device Errors"=w258:cluster{"code":i32, "Text":string}[])  [unwired: 7 in, 1 out]
          }
          event "Get Trigger Rate": Value Change {
            n125 = event-data() -> ()  [unwired: 1 in, 1 out]
            n126 = call "Get Trigger Rate.vi"("VISA resource name"=w263) -> ("error out"=w264:errorcluster, "Trigger Rate [Hz]"=→"Current Trigger Rate [Hz]":dbl, "Device Errors"=w262:cluster{"code":i32, "Text":string}[])  [unwired: 7 in, 1 out]
          }
          event "Set Trigger Rate [Hz]": Value Change {
            n127 = event-data() -> ()  [unwired: 1 in, 1 out]
            n128 = call "Set Trigger Rate.vi"("Trigger Rate (1e3) [Hz]"="Set Trigger Rate [Hz]", "VISA resource name"=w267) -> ("error out"=w268:errorcluster, "Device Errors"=w266:cluster{"code":i32, "Text":string}[])  [unwired: 7 in, 1 out]
          }
          event "Get Trigger Source": Value Change {
            n129 = event-data() -> ()  [unwired: 1 in, 1 out]
            n130 = call "Get Trigger Source.vi"("VISA resource name"=w271) -> ("error out"=w272:errorcluster, "Trigger Source"=→"Current Trigger Source":i32, "Device Errors"=w270:cluster{"code":i32, "Text":string}[])  [unwired: 7 in, 1 out]
          }
          event "Set Trigger Source": Value Change {
            n131 = event-data() -> ()  [unwired: 1 in, 1 out]
            n132 = call "Set Trigger Source.vi"("Trigger Source (Internal)"="Set Trigger Source", "VISA resource name"=w275) -> ("error out"=w276:errorcluster, "Device Errors"=w274:cluster{"code":i32, "Text":string}[])  [unwired: 7 in, 1 out]
          }
          event "Get Burst Count": Value Change {
            n133 = event-data() -> ()  [unwired: 1 in, 1 out]
            n134 = call "Get Burst Count.vi"("VISA resource name"=w279) -> ("error out"=w280:errorcluster, "Burst Count"=→"Current Burst Count":i32, "Device Errors"=w278:cluster{"code":i32, "Text":string}[])  [unwired: 7 in, 1 out]
          }
          event "Set Burst Count": Value Change {
            n135 = event-data() -> ()  [unwired: 1 in, 1 out]
            n136 = call "Set Burst Count.vi"("Burst Count"="Set Burst Count", "VISA resource name"=w283) -> ("error out"=w284:errorcluster, "Device Errors"=w282:cluster{"code":i32, "Text":string}[])  [unwired: 7 in, 1 out]
          }
          event "Get Burst Delay": Value Change {
            n137 = event-data() -> ()  [unwired: 1 in, 1 out]
            n138 = call "Get Burst Delay.vi"("VISA resource name"=w287) -> ("error out"=w288:errorcluster, "Burst Delay [s]"=→"Current Burst Delay [s]":dbl, "Device Errors"=w286:cluster{"code":i32, "Text":string}[])  [unwired: 7 in, 1 out]
          }
          event "Set Burst Delay [s]": Value Change {
            n139 = event-data() -> ()  [unwired: 1 in, 1 out]
            n140 = call "Set Burst Delay.vi"("Burst Delay [s]"="Set Burst Delay [s]", "VISA resource name"=w291) -> ("error out"=w292:errorcluster, "Device Errors"=w290:cluster{"code":i32, "Text":string}[])  [unwired: 7 in, 1 out]
          }
          event "Get Burst Mode": Value Change {
            n141 = event-data() -> ()  [unwired: 1 in, 1 out]
            n142 = call "Get Burst Mode.vi"("VISA resource name"=w295) -> ("error out"=w296:errorcluster, "Burst Mode enabled?"=→"Burst Mode enabled?":bool, "Device Errors"=w294:cluster{"code":i32, "Text":string}[])  [unwired: 7 in, 1 out]
          }
          event "Set Burst Mode": Value Change {
            n143 = event-data() -> ()  [unwired: 1 in, 1 out]
            n144 = call "Set Burst Mode.vi"("Enable Burst Mode"="Set Burst Mode", "VISA resource name"=w299) -> ("error out"=w300:errorcluster, "Device Errors"=w298:cluster{"code":i32, "Text":string}[])  [unwired: 7 in, 1 out]
          }
          event "Get Burst Period": Value Change {
            n145 = event-data() -> ()  [unwired: 1 in, 1 out]
            n146 = call "Get Burst Period.vi"("VISA resource name"=w303) -> ("error out"=w304:errorcluster, "Burst Period [s]"=→"Current Burst Period [s]":dbl, "Device Errors"=w302:cluster{"code":i32, "Text":string}[])  [unwired: 7 in, 1 out]
          }
          event "Set Burst Period [s]": Value Change {
            n147 = event-data() -> ()  [unwired: 1 in, 1 out]
            n148 = call "Set Burst Period.vi"("Burst Period [s] (1E-7)"="Set Burst Period [s]", "VISA resource name"=w307) -> ("error out"=w308:errorcluster, "Device Errors"=w306:cluster{"code":i32, "Text":string}[])  [unwired: 7 in, 1 out]
          }
          event "Get Burst T0 Config": Value Change {
            n149 = event-data() -> ()  [unwired: 1 in, 1 out]
            n150 = call "Get Burst T0 Config.vi"("VISA resource name"=w311) -> ("error out"=w312:errorcluster, "Burst T0 Config enabled?"=→"Burst T0 Config enabled?":bool, "Device Errors"=w310:cluster{"code":i32, "Text":string}[])  [unwired: 7 in, 1 out]
          }
          event "Set Burst T0 Config": Value Change {
            n151 = event-data() -> ()  [unwired: 1 in, 1 out]
            n152 = call "Set Burst T0 Config.vi"("Enable Burst T0 Config"="Set Burst T0 Config", "VISA resource name"=w315) -> ("error out"=w316:errorcluster, "Device Errors"=w314:cluster{"code":i32, "Text":string}[])  [unwired: 7 in, 1 out]
          }
          event "Step Burst Count": Value Change {
            n153 = event-data() -> ()  [unwired: 1 in, 1 out]
            n154 = call "Step Burst Count.vi"("Step up? (false)"="Burst Count Step Direction", "VISA resource name"=w319) -> ("error out"=w320:errorcluster, "Device Errors"=w318:cluster{"code":i32, "Text":string}[])  [unwired: 7 in, 1 out]
          }
          event "Get Burst Count Step Size": Value Change {
            n155 = event-data() -> ()  [unwired: 1 in, 1 out]
            n156 = call "Get Step Size Burst Count.vi"("VISA resource name"=w323) -> ("error out"=w324:errorcluster, "Step Size Burst Count"=→"Burst Count Step Size":i32, "Device Errors"=w322:cluster{"code":i32, "Text":string}[])  [unwired: 7 in, 1 out]
          }
          event "Set Burst Count Step Size": Value Change {
            n157 = event-data() -> ()  [unwired: 1 in, 1 out]
            n158 = call "Set Step Size Burst Count.vi"("Step Size Burst Count"="Set Burst Count Step Size", "VISA resource name"=w327) -> ("error out"=w328:errorcluster, "Device Errors"=w326:cluster{"code":i32, "Text":string}[])  [unwired: 7 in, 1 out]
          }
          event "Step Burst Delay": Value Change {
            n159 = event-data() -> ()  [unwired: 1 in, 1 out]
            n160 = call "Step Burst Delay.vi"("Step up? (false)"="Burst Delay Step Direction", "VISA resource name"=w331) -> ("error out"=w332:errorcluster, "Device Errors"=w330:cluster{"code":i32, "Text":string}[])  [unwired: 7 in, 1 out]
          }
          event "Get Burst Delay Step Size": Value Change {
            n161 = event-data() -> ()  [unwired: 1 in, 1 out]
            n162 = call "Get Step Size Burst Delay.vi"("VISA resource name"=w335) -> ("error out"=w336:errorcluster, "Step Size Burst Delay [s]"=→"Burst Delay Step Size [s]":dbl, "Device Errors"=w334:cluster{"code":i32, "Text":string}[])  [unwired: 7 in, 1 out]
          }
          event "Set Burst Delay Step Size [s]": Value Change {
            n163 = event-data() -> ()  [unwired: 1 in, 1 out]
            n164 = call "Set Step Size Burst Delay.vi"("Step Size Burst Delay [s]"="Set Burst Delay Step Size [s]", "VISA resource name"=w339) -> ("error out"=w340:errorcluster, "Device Errors"=w338:cluster{"code":i32, "Text":string}[])  [unwired: 7 in, 1 out]
          }
          event "Step Burst Period": Value Change {
            n165 = event-data() -> ()  [unwired: 1 in, 1 out]
            n166 = call "Step Burst Period.vi"("Step up? (false)"="Burst Period Step Direction", "VISA resource name"=w343) -> ("error out"=w344:errorcluster, "Device Errors"=w342:cluster{"code":i32, "Text":string}[])  [unwired: 7 in, 1 out]
          }
          event "Get Burst Period Step Size": Value Change {
            n167 = event-data() -> ()  [unwired: 1 in, 1 out]
            n168 = call "Get Step Size Burst Period.vi"("VISA resource name"=w347) -> ("error out"=w348:errorcluster, "Step Size Burst Period [s]"=→"Burst Period Step Size [Hz]":dbl, "Device Errors"=w346:cluster{"code":i32, "Text":string}[])  [unwired: 7 in, 1 out]
          }
          event "Set Burst Period Step Size [Hz]": Value Change {
            n169 = event-data() -> ()  [unwired: 1 in, 1 out]
            n170 = call "Set Step Size Burst Period.vi"("Step Size Burst Period [s]"="Set Burst Period Step Size [Hz]", "VISA resource name"=w351) -> ("error out"=w352:errorcluster, "Device Errors"=w350:cluster{"code":i32, "Text":string}[])  [unwired: 7 in, 1 out]
          }
          event Value Change {
            n171 = event-data() -> ()  [unwired: 1 in, 1 out]
            n172 = call "Get Delay.vi"("Channel (T0)"="Get Delay Channel", "VISA resource name"=w357) -> ("error out"=w358:errorcluster, "Delay [s]"=→"Current Delay [s]":dbl, "relative to"=→"currently relative to":T6, "Device Errors"=w356:cluster{"code":i32, "Text":string}[])  [unwired: 5 in, 1 out]
          }
          event "Set: Delay [s]": Value Change {
            n173 = event-data() -> ()  [unwired: 1 in, 1 out]
            n174 = call "Set Delay.vi"("Delay (0) [s]"="Set: Delay [s]", "relative to (T0)"="Set: relative to", "Channel (T0)"="Set Delay Channel", "VISA resource name"=w363) -> ("error out"=w364:errorcluster, "Device Errors"=w362:cluster{"code":i32, "Text":string}[])  [unwired: 5 in, 1 out]
          }
          event Value Change {
            n175 = event-data() -> ()  [unwired: 1 in, 1 out]
            n176 = call "Get Level Amplitude.vi"("Output BNC (T0)"="Get Level Amplitude Output BNC", "VISA resource name"=w368) -> ("error out"=w369:errorcluster, "Level Amplitue [V]"=→"Current Level Amplitude Output BNC [V]":dbl, "Device Errors"=w367:cluster{"code":i32, "Text":string}[])  [unwired: 6 in, 1 out]
          }
          event "Set: Level Amplitude [V]": Value Change {
            n177 = event-data() -> ()  [unwired: 1 in, 1 out]
            n178 = call "Set Level Amplitude.vi"("Level Amplitude (0) [V]"="Set: Level Amplitude [V]", "Output BNC (T0)"="Set Level Amplitude Output BNC", "VISA resource name"=w373) -> ("error out"=w374:errorcluster, "Device Errors"=w372:cluster{"code":i32, "Text":string}[])  [unwired: 6 in, 1 out]
          }
          event Value Change {
            n179 = event-data() -> ()  [unwired: 1 in, 1 out]
            n180 = call "Get Link Channel.vi"("Channel (A)"="Get Link of Channel", "VISA resource name"=w378) -> ("error out"=w379:errorcluster, "linked to"=→"currently linked to":T6, "Device Errors"=w377:cluster{"code":i32, "Text":string}[])  [unwired: 6 in, 1 out]
          }
          event Value Change {
            n181 = event-data() -> ()  [unwired: 1 in, 1 out]
            n182 = call "Set Link Channel.vi"("Link to (B)"="Set: Link to", "Channel (A)"="Set Link of Channel", "VISA resource name"=w383) -> ("error out"=w384:errorcluster, "Device Errors"=w382:cluster{"code":i32, "Text":string}[])  [unwired: 6 in, 1 out]
          }
          event Value Change {
            n183 = event-data() -> ()  [unwired: 1 in, 1 out]
            n184 = call "Get Level Offset.vi"("Output BNC (T0)"="Get Level Offset of Output", "VISA resource name"=w388) -> ("error out"=w389:errorcluster, "Level Offset [V]"=→"Current Level Offset [V]":dbl, "Device Errors"=w387:cluster{"code":i32, "Text":string}[])  [unwired: 6 in, 1 out]
          }
          event Value Change {
            n185 = event-data() -> ()  [unwired: 1 in, 1 out]
            n186 = call "Set Level Offset.vi"("Level Offset (0) [V]"="Set Level Offset [V]", "Output BNC (T0)"="Set Level Offset of Output", "VISA resource name"=w393) -> ("error out"=w394:errorcluster, "Device Errors"=w392:cluster{"code":i32, "Text":string}[])  [unwired: 6 in, 1 out]
          }
          event Value Change {
            n187 = event-data() -> ()  [unwired: 1 in, 1 out]
            n188 = call "Get Level Polarity.vi"("Output BNC (AB)"="Get Level Polarity of Output", "VISA resource name"=w398) -> ("error out"=w399:errorcluster, "Polarity"=→"Current Polarity":T12, "Device Errors"=w397:cluster{"code":i32, "Text":string}[])  [unwired: 6 in, 1 out]
          }
          event Value Change {
            n189 = event-data() -> ()  [unwired: 1 in, 1 out]
            n190 = call "Set Level Polarity.vi"("Polarity (positive)"="Polarity to be set", "Output BNC (AB)"="Set Level Polarity of Output", "VISA resource name"=w403) -> ("error out"=w404:errorcluster, "Device Errors"=w402:cluster{"code":i32, "Text":string}[])  [unwired: 6 in, 1 out]
          }
          event "Step Delay": Value Change {
            n191 = event-data() -> ()  [unwired: 1 in, 1 out]
            n192 = call "Step Delay.vi"("Step up? (false)"="Delay Step Direction", "Channel (T0)"="Channel Step Delay", "VISA resource name"=w408) -> ("error out"=w409:errorcluster, "Device Errors"=w407:cluster{"code":i32, "Text":string}[])  [unwired: 6 in, 1 out]
          }
          event "Get Step Size Delay": Value Change {
            n193 = event-data() -> ()  [unwired: 1 in, 1 out]
            n194 = property on="Channel Step Delay" class="Ring (strict)"() -> (error out=w411:errorcluster, "Value"=w412:T14)  [unwired: 2 in, 1 out]
            n195 = call "Get Step Size Delay.vi"("error in (no error)"=w411, "Channel (T0)"=w412, "VISA resource name"=w414) -> ("error out"=w415:errorcluster, "Step Size Delay [s]"=→"Step Size Delay [s]":dbl, "Device Errors"=w413:cluster{"code":i32, "Text":string}[])  [unwired: 5 in, 1 out]
          }
          event "Set Step Size Delay [s]": Value Change {
            n196 = event-data() -> ()  [unwired: 1 in, 1 out]
            n197 = property on="Channel Step Delay" class="Ring (strict)"() -> (error out=w417:errorcluster, "Value"=w418:T14)  [unwired: 2 in, 1 out]
            n198 = call "Set Step Size Delay.vi"("error in (no error)"=w417, "Step Size Delay (0) [s]"="Set Step Size Delay [s]", "Channel (T0)"=w418, "VISA resource name"=w420) -> ("error out"=w421:errorcluster, "Device Errors"=w419:cluster{"code":i32, "Text":string}[])  [unwired: 5 in, 1 out]
          }
          event "Step Level Amplitude": Value Change {
            n199 = event-data() -> ()  [unwired: 1 in, 1 out]
            n200 = call "Step Level Amplitude.vi"("Step up? (false)"="Level Amplitude Step Direction", "Output BNC (T0)"="Output BNC Step Level Ampitude", "VISA resource name"=w425) -> ("error out"=w426:errorcluster, "Device Errors"=w424:cluster{"code":i32, "Text":string}[])  [unwired: 6 in, 1 out]
          }
          event "Get Step Size Level Amplitude": Value Change {
            n201 = event-data() -> ()  [unwired: 1 in, 1 out]
            n202 = property on="Output BNC Step Level Ampitude" class="Ring (strict)"() -> (error out=w428:errorcluster, "Value"=w427:T15)  [unwired: 2 in, 1 out]
            n203 = call "Get Step Size Level Amplitude.vi"("error in (no error)"=w428, "Output BNC (T0)"=w427, "VISA resource name"=w431) -> ("error out"=w432:errorcluster, "Step Size Level Amplitue [V]"=→"Step Size  Level Amplitude [V]":dbl, "Device Errors"=w430:cluster{"code":i32, "Text":string}[])  [unwired: 5 in, 1 out]
          }
          event "Set Step Size L-Amplitude [V]": Value Change {
            n204 = event-data() -> ()  [unwired: 1 in, 1 out]
            n205 = property on="Output BNC Step Level Ampitude" class="Ring (strict)"() -> (error out=w435:errorcluster, "Value"=w434:T15)  [unwired: 2 in, 1 out]
            n206 = call "Set Step Size Level Amplitude.vi"("error in (no error)"=w435, "Step Size Level Amplitude (0) [V]"="Set Step Size L-Amplitude [V]", "Output BNC (T0)"=w434, "VISA resource name"=w437) -> ("error out"=w438:errorcluster, "Device Errors"=w436:cluster{"code":i32, "Text":string}[])  [unwired: 5 in, 1 out]
          }
          event "Step Level Offset": Value Change {
            n207 = event-data() -> ()  [unwired: 1 in, 1 out]
            n208 = call "Step Level Offset.vi"("Step up? (false)"="Level Offset Step Direction", "Output BNC (T0)"="Output BNC Level Offset", "VISA resource name"=w442) -> ("error out"=w443:errorcluster, "Device Errors"=w441:cluster{"code":i32, "Text":string}[])  [unwired: 6 in, 1 out]
          }
          event "Get Step Size Level Offset": Value Change {
            n209 = event-data() -> ()  [unwired: 1 in, 1 out]
            n210 = property on="Output BNC Level Offset" class="Ring (strict)"() -> (error out=w445:errorcluster, "Value"=w444:T15)  [unwired: 2 in, 1 out]
            n211 = call "Get Step Size Level Offset.vi"("error in (no error)"=w445, "Output BNC (T0)"=w444, "VISA resource name"=w448) -> ("error out"=w449:errorcluster, "Step Size Level Offset [V]"=→"Step Size  Level Offset [V]":dbl, "Device Errors"=w447:cluster{"code":i32, "Text":string}[])  [unwired: 5 in, 1 out]
          }
          event "Set Step Size L-Offset [V]": Value Change {
            n212 = event-data() -> ()  [unwired: 1 in, 1 out]
            n213 = property on="Output BNC Level Offset" class="Ring (strict)"() -> (error out=w452:errorcluster, "Value"=w451:T15)  [unwired: 2 in, 1 out]
            n214 = call "Set Step Size Level Offset.vi"("error in (no error)"=w452, "Step Size Level Offset (0) [V]"="Set Step Size L-Offset [V]", "Output BNC (T0)"=w451, "VISA resource name"=w454) -> ("error out"=w455:errorcluster, "Device Errors"=w453:cluster{"code":i32, "Text":string}[])  [unwired: 5 in, 1 out]
          }
          event "Get Ethernet MAC Address": Value Change {
            n215 = event-data() -> ()  [unwired: 1 in, 1 out]
            n216 = call "MAC Address.vi"("VISA resource name"=w458) -> ("error out"=w459:errorcluster, "Ethernet MAC address"=→"Ethernet MAC address":string, "Device Errors"=w457:cluster{"code":i32, "Text":string}[])  [unwired: 7 in, 1 out]
          }
          event "Get Ethernet Physical Layer Config": Value Change {
            n217 = event-data() -> ()  [unwired: 1 in, 1 out]
            n218 = call "Get Ethernet Physical Layer Configuration.vi"("Configuration (Enable/disable Auto-negotiation of link speed)"="Get Ethernet Physical Layer Config", "VISA resource name"=w463) -> ("error out"=w464:errorcluster, "Value"=→"Ethernet Physical Layer Config":bool, "Device Errors"=w462:cluster{"code":i32, "Text":string}[])  [unwired: 6 in, 1 out]
          }
          event "Set Ethernet Physical Layer Config", "Ethernet Physical Layer Config to set": Value Change {
            n219 = event-data() -> ()  [unwired: 1 in, 1 out]
            n220 = call "Set Ethernet Physical Layer Configuration.vi"("Value"="Ethernet Physical Layer Config to set", "Configuration (Enable/disable Auto-negotiation of link speed)"="Set Ethernet Physical Layer Config", "VISA resource name"=w468) -> ("error out"=w469:errorcluster, "Device Errors"=w467:cluster{"code":i32, "Text":string}[])  [unwired: 6 in, 1 out]
          }
          event "Get Interface Config": Value Change {
            n221 = event-data() -> ()  [unwired: 1 in, 1 out]
            n222 = call "Get Interface Configuration.vi"("Configuration Parameter (RS-232 Enable/Disable)"="Get Interface Config", "VISA resource name"=w473) -> ("error out"=w474:errorcluster, "Value"=→"Current Interface Config Value":string, "Device Errors"=w472:cluster{"code":i32, "Text":string}[])  [unwired: 6 in, 1 out]
          }
          event "Set Interface Config": Value Change {
            n223 = event-data() -> ()  [unwired: 1 in, 1 out]
            n224 = call "Set Interface Configuration.vi"("Value (0)"="Interface Config Value to set", "Configuration Parameter (RS-232 Enable/Disable)"="Set Interface Config", "VISA resource name"=w478) -> ("error out"=w479:errorcluster, "Device Errors"=w477:cluster{"code":i32, "Text":string}[])  [unwired: 6 in, 1 out]
          }
          event "Interface to reset": Value Change {
            n225 = event-data() -> ()  [unwired: 1 in, 1 out]
            n226 = call "Interface Reset.vi"("Interface"="Interface to reset", "VISA resource name"=w482) -> ("error out"=w483:errorcluster, "Device Errors"=w481:cluster{"code":i32, "Text":string}[])  [unwired: 7 in, 1 out]
          }
          event "Set Local": Value Change {
            n227 = event-data() -> ()  [unwired: 1 in, 1 out]
            n228 = call "Local.vi"("VISA resource name"=w485) -> ("error out"=w486:errorcluster, "Device Errors"=w484:cluster{"code":i32, "Text":string}[])  [unwired: 8 in, 1 out]
          }
          event "Lock": Value Change {
            n229 = event-data() -> ()  [unwired: 1 in, 1 out]
            n230 = call "Lock.vi"("VISA resource name"=w489) -> ("error out"=w490:errorcluster, "locked?"=→"locked?":bool, "Device Errors"=w488:cluster{"code":i32, "Text":string}[])  [unwired: 7 in, 1 out]
          }
          event "Set Remote": Value Change {
            n231 = event-data() -> ()  [unwired: 1 in, 1 out]
            n232 = call "Remote.vi"("VISA resource name"=w492) -> ("error out"=w493:errorcluster, "Device Errors"=w491:cluster{"code":i32, "Text":string}[])  [unwired: 8 in, 1 out]
          }
          event "Unlock": Value Change {
            n233 = event-data() -> ()  [unwired: 1 in, 1 out]
            n234 = call "Unlock.vi"("VISA resource name"=w496) -> ("error out"=w497:errorcluster, "unlocked?"=→"unlocked?":bool, "Device Errors"=w495:cluster{"code":i32, "Text":string}[])  [unwired: 7 in, 1 out]
          }
          event "i", "j", "k": Value Change {
            n235 = event-data() -> ()  [unwired: 1 in, 1 out]
            n236 = call "Interface Terminator.vi"("k (0)"="k", "j (0)"="j", "i (0)"="i", "VISA resource name"=w502) -> ("error out"=w503:errorcluster, "Device Errors"=w501:cluster{"code":i32, "Text":string}[])  [unwired: 5 in, 1 out]
          }
          event "Get Revision": Value Change {
            n237 = event-data() -> ()  [unwired: 1 in, 1 out]
            n238 = call "Revision Query.vi"("VISA resource name"=w507) -> ("error out"=w508:errorcluster, "Instrument Firmware Revision"=→"Instrument Firmware Rev":string, "Instrument Driver Revision"=→"Instrument Driver Revision":string, "Device Errors"=w506:cluster{"code":i32, "Text":string}[])  [unwired: 6 in, 1 out]
          }
          event "stop": Value Change {
            n239 = event-data() -> ()  [unwired: 1 in, 1 out]
            n240 = call "Close.vi"("VISA resource name"=w511) -> ("error out"=w512:errorcluster, "Device Errors"=w509:cluster{"code":i32, "Text":string}[])  [unwired: 9 in]
          }
        }
        n241 = local write "error out"(w11) -> ()
        n242 = local write "Device Errors"(w10) -> ()
      }
    }
    frame Error {
    }
  }
